vi "Get SettingsXML from Path.vi"(10 "Rev Path":path) -> (0 "XML File Found":bool, 2 "Rev Path out":path, 3 "Controls":T1={"Confocal Controls"={"Channel Selection"=enum."A", "Pixel Count"={"Pixels in X"=512, "Pixels in Y"=512}, "Field Size"=174.0, "Frames"=0, "Averaging"=FALSE, "Alignment"=0.0, "Scan Mode"=TRUE, "Gain"={"Gain A"=0, "Gain B"=0}, "Enable PMTs"={"A"=TRUE, "B"=TRUE}, "Voltage Range"={"Range A"=10, "Range B"=10}, "Multi Frame Count"=0.0, "Trigger Mode"=2.0, "Real Time Averaging"=TRUE, "PFOV"=0.0, "MicronsPerPx"=0.0}, "iFlex Control"={"Power 561"=0.0, "Power 488"=0.0, "Global Shutter"=FALSE, "561 Shutter"=FALSE}, "PIFOC Settings"={"PIFOC Position (mm) [SET]"=0.0, "PIFOC Position\n(um) [ACT]"=0.0087, "last command"=""}, "PinSelector"=6.0, "Manlight Controls"={"Manlight Power"=0.0, "Open Serial"=FALSE, "VISA Refnum"=""}, "Exp Params"={"Experiment Type"="2D Snapshot", "Experiment Name"="Experiment_1", "ExpPath"=path "E:/Data", "TSFrames"=1000, "TSfps"=1000, "ZTSFrames"=1000, "ZTSdt"=1, "Streaming"=FALSE, "Z Stack Settings"={"Start"=0.0, "Step Size"=0.1, "Finish"=1.0}, "total images"=1, "tdms ref"=refnum, "frame #"=0, "images per stack"=1, "total stacks"=1, "period"=1, "PI MVR Increment"=""}} {"Exp Params"."period" min=1; "Exp Params"."total stacks" min=1; "Exp Params"."images per stack" min=1; "Exp Params"."total images" min=1; "Exp Params"."Z Stack Settings"."Start" min=0.0 max=100.0 step=0.1; "Exp Params"."Z Stack Settings"."Step Size" min=0.1 max=100.0 step=0.1; "Exp Params"."Z Stack Settings"."Finish" min=0.0 max=100.0 step=0.1; "Exp Params"."TSFrames" min=1 step=1; "Exp Params"."ZTSdt" min=1 step=1; "Exp Params"."ZTSFrames" min=2 step=1; "Exp Params"."TSfps" min=1 max=1000 step=1; "Manlight Controls"."Manlight Power" min=0.0 max=10.0 step=0.1 scale=0.0..10.0; "PinSelector" items=["25", "30", "35", "40", "45", "50", "60", "70", "80", "90", "100", "125", "200", "300", "1000", "2000"]; "PIFOC Settings"."PIFOC Position\n(um) [ACT]" format="%.2f"; "PIFOC Settings"."PIFOC Position (mm) [SET]" min=0.0 max=100.0 step=0.1 scale=0.0..100.0; "iFlex Control"."Power 561" min=12.5 max=100.0 step=0.1 scale=0.0..100.0; "iFlex Control"."Power 488" min=30.0 max=100.0 step=0.1 scale=0.0..100.0; "Confocal Controls"."Field Size" min=5.0 max=255.0 step=1.0 scale=5.0..255.0; "Confocal Controls"."PFOV" min=1.0 max=300.0 step=0.1; "Confocal Controls"."MicronsPerPx" min=0.01 step=0.01 format="%.2f"; "Confocal Controls"."Gain"."Gain B" min=1 max=100 step=1; "Confocal Controls"."Gain"."Gain A" min=1 max=100 step=1; "Confocal Controls"."Voltage Range"."Range B" items=["100mV"=5, "200mV"=6, "400mV"=7, "1V"=10, "2V"=11, "4V"=12]; "Confocal Controls"."Voltage Range"."Range A" items=["100mV"=5, "200mV"=6, "400mV"=7, "1V"=10, "2V"=11, "4V"=12]; "Confocal Controls"."Pixel Count"."Pixels in Y" items=["32"=32, "64"=64, "128"=128, "256"=256, "512"=512, "1024"=1024, "2048"=2048]; "Confocal Controls"."Pixel Count"."Pixels in X" items=["32"=32, "64"=64, "128"=128, "256"=256, "512"=512, "1024"=1024, "2048"=2048]})   [LabVIEW 2020]
uses:
  _Controls/All Controls For Saving.ctl
  _Controls/Confocal Controls.ctl
  _Controls/iFlex.ctl
  _Controls/PIFOC Position.ctl
  _Controls/Manlight Controls.ctl
  _Controls/Exp Params.ctl
  <vilib>/Utility/xml.llb/Read From XML File(string).vi
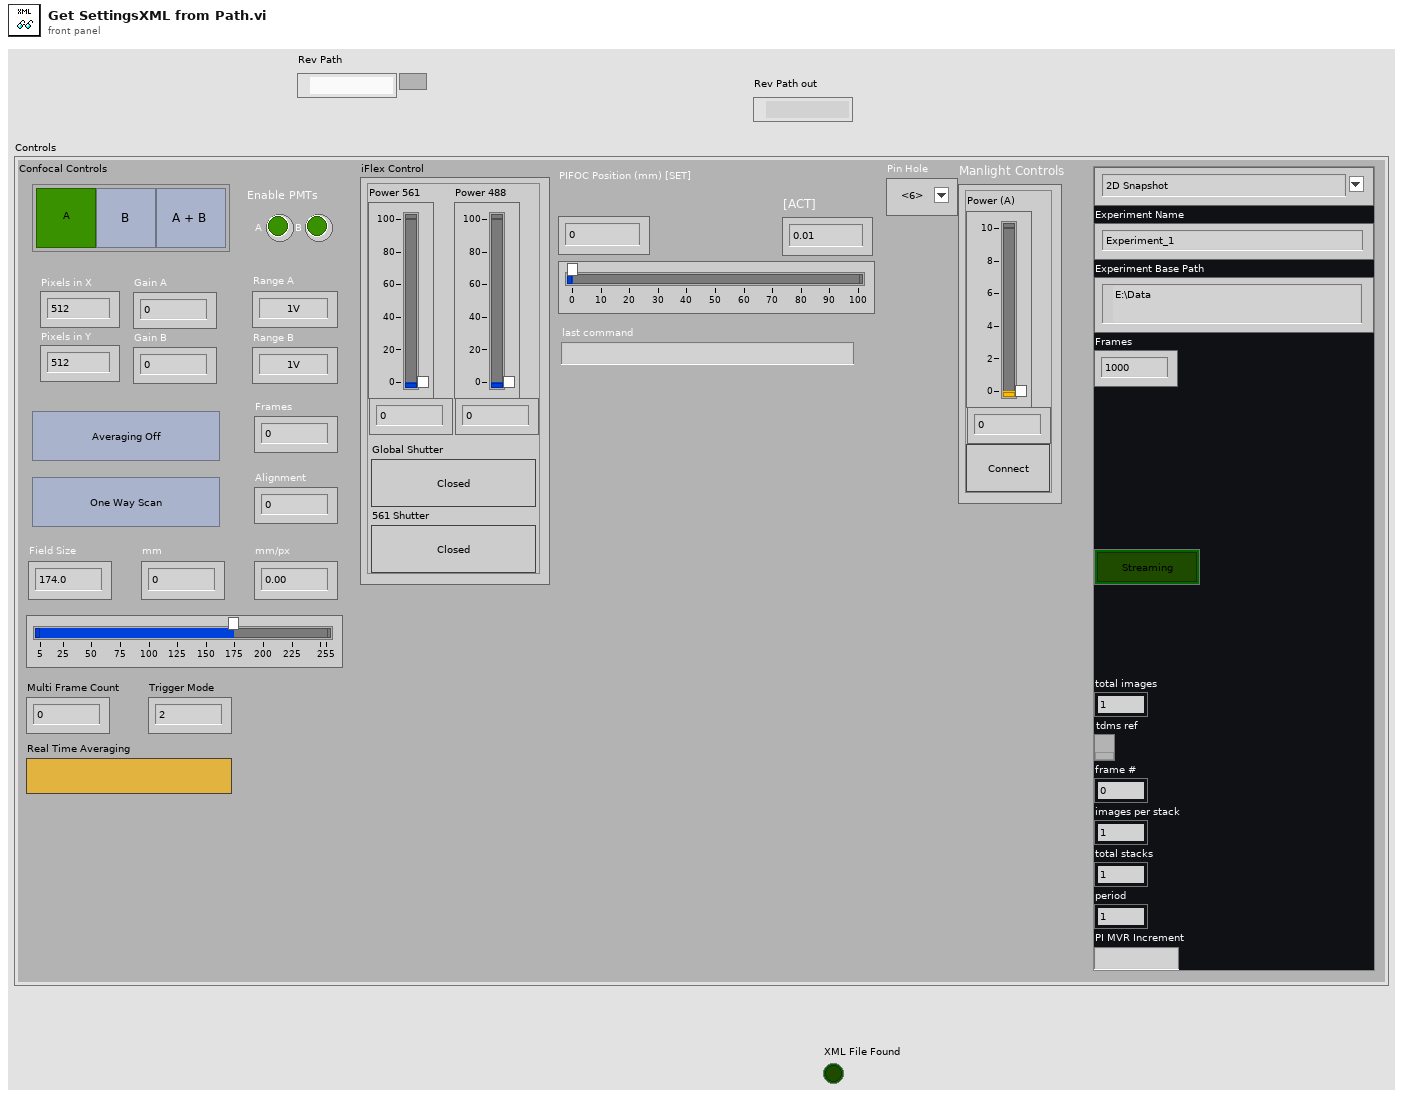
[diagram p1: front panel]
types:
  T1 = typedef "All Controls For Saving.ctl" = cluster{"Confocal Controls":T2, "iFlex Control":T3, "PIFOC Settings":T4, "PinSelector":dbl, "Manlight Controls":T5, "Exp Params":T6}
  T2 = typedef "Confocal Controls.ctl" = cluster{"Channel Selection":enum32{"A", "B", "AB"}, "Pixel Count":cluster{"Pixels in X":u32, "Pixels in Y":u32}, "Field Size":dbl, "Frames":u8, "Averaging":bool, "Alignment":dbl, "Scan Mode":bool, "Gain":cluster{"Gain A":u8, "Gain B":u8}, "Enable PMTs":cluster{"A":bool, "B":bool}, "Voltage Range":cluster{"Range A":u16, "Range B":u16}, "Multi Frame Count":dbl, "Trigger Mode":dbl, "Real Time Averaging":bool, "PFOV":dbl, "MicronsPerPx":dbl}
  T3 = typedef "iFlex.ctl" = cluster{"Power 561":dbl, "Power 488":dbl, "Global Shutter":bool, "561 Shutter":bool}
  T4 = typedef "PIFOC Position.ctl" = cluster{"PIFOC Position (mm) [SET]":dbl, "PIFOC Position\n(um) [ACT]":dbl, "last command":string}
  T5 = typedef "Manlight Controls.ctl" = cluster{"Manlight Power":dbl, "Open Serial":bool, "VISA Refnum":refnum<visa-resource-name>}
  T6 = typedef "Exp Params.ctl" = cluster{"Experiment Type":string, "Experiment Name":string, "ExpPath":path, "TSFrames":i32, "TSfps":i32, "ZTSFrames":i32, "ZTSdt":i32, "Streaming":bool, "Z Stack Settings":cluster{"Start":dbl, "Step Size":dbl, "Finish":dbl}, "total images":i32, "tdms ref":refnum<k34>, "frame #":i64, "images per stack":i32, "total stacks":i32, "period":i32, "PI MVR Increment":string}
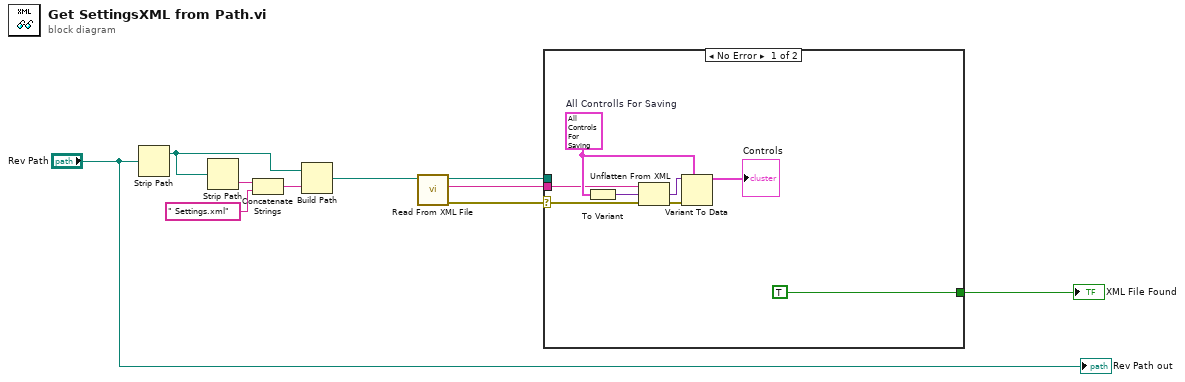
[diagram p0: block diagram]
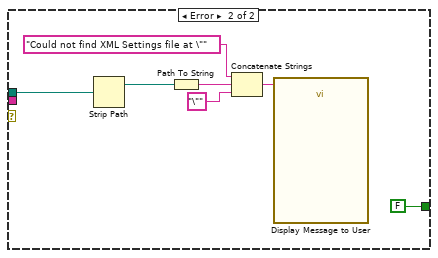
[diagram p2: hidden frame]
diagram:
  n1 = Strip Path(path="Rev Path") -> (stripped path=w4:path)  [unwired: 1 out]
  n2 = Strip Path(path=w4) -> (name=w7:string)  [unwired: 1 out]
  n3 = Concatenate Strings(w7, " Settings.xml" ("string")) -> (w9:string)
  n4 = Build Path(base path=w4, name or relative path=w9) -> (appended path=w10:path)
  n5 = call-poly <vilib>:"Read From XML File.vi"("XML File Path"=w10) -> ("error out"=w3:errorcluster, "XML Elements"=w6:string, "XML File Path(duplicate)"=w2:path)  [unwired: 8 in]
  n6 = case shown="No Error" w3 {
    selector: w3 -> [w13 _]
    tunnel: w6 -> [w17 _]
    tunnel: w2 -> [_ w20]
    tunnel: [TRUE ("OK") FALSE ("OK")] -> w1
    frame No Error {
      w18 = T1 {"Confocal Controls"={"Channel Selection"=enum."A", "Pixel Count"={"Pixels in X"=512, "Pixels in Y"=512}, "Field Size"=0.0, "Frames"=0, "Averaging"=FALSE, "Alignment"=0.0, "Scan Mode"=FALSE, "Gain"={"Gain A"=0, "Gain B"=0}, "Enable PMTs"={"A"=FALSE, "B"=FALSE}, "Voltage Range"={"Range A"=10, "Range B"=10}, "Multi Frame Count"=0.0, "Trigger Mode"=0.0, "Real Time Averaging"=FALSE, "PFOV"=0.0, "MicronsPerPx"=0.0}, "iFlex Control"={"Power 561"=0.0, "Power 488"=0.0, "Global Shutter"=FALSE, "561 Shutter"=FALSE}, "PIFOC Settings"={"PIFOC Position (mm) [SET]"=0.0, "PIFOC Position\n(um) [ACT]"=0.0087, "last command"=""}, "PinSelector"=6.0, "Manlight Controls"={"Manlight Power"=0.0, "Open Serial"=FALSE, "VISA Refnum"=""}, "Exp Params"={"Experiment Type"="2D Snapshot", "Experiment Name"="Experiment_1", "ExpPath"=path "E:/Data", "TSFrames"=1000, "TSfps"=1000, "ZTSFrames"=1000, "ZTSdt"=1, "Streaming"=FALSE, "Z Stack Settings"={"Start"=0.0, "Step Size"=0.1, "Finish"=1.0}, "total images"=1, "tdms ref"=refnum, "frame #"=0, "images per stack"=1, "total stacks"=1, "period"=1, "PI MVR Increment"=""}}  # All Controlls For Saving
      n7 = To Variant(anything=w18) -> (Variant=w16:variant)
      n8 = Unflatten From XML(xml string=w17, type=w16, error in (no error)=w13) -> (value=w15:variant, error out=w14:errorcluster)
      n9 = Variant To Data(error in=w14, type=w18, Variant=w15) -> (data=→"Controls":T1)  [unwired: 1 out]
    }
    frame Error {
      n10 = Strip Path(path=w20) -> (stripped path=w22:path)  [unwired: 1 out]
      n11 = Path To String(path=w22) -> (string=w25:string)
      n12 = Concatenate Strings("Could not find XML Settings file at \"" ("string"), w25, "\"" ("string")) -> (w23:string)
      n13 = call "Display Message to User"("Message"=w23) -> ()  [unwired: 9 in, 2 out]
    }
  }
  "XML File Found" <- w1
  "Rev Path out" <- "Rev Path"
